vi "NMRvmefull7.vi"() -> ()   [LabVIEW 2013]
uses:
  <vilib>/Utility/file.llb/Read From Spreadsheet File (DBL).vi
  <vilib>/Analysis/NI_AALBase.lvlib
panel:
  out "Telnet error out":errorcluster
  in  "Real/quad Q curve":bool=TRUE
  out "Temperature (C)":dbl(graph)=23.38
  out "+3V supply":dbl=0.005 format="%_4g"
  out "Temp (C)":dbl=23.38 format="%_4g"
  in  "RemovePed":bool=TRUE
  in  "IF / LOG Det":bool
  in  "Q curve file":string="realback213.txt"
  out "File name 2":string="C:\\users\\plm\\Desktop\\rssmt\\realback213.txt"
  in  "AutoBaseline":bool=TRUE
  out "RF OK":bool=TRUE
  out "Peak area (V-MHz)":sgl=0.042041864 format="%.5f"
  in  "Gauss Fit":bool=TRUE
  out "NMR Graph + Fit":cluster{cluster{dbl, "Numeric":dbl}[]}[](graph)=[{[{212.6, "Numeric"=-0.015064761904761914}, {212.60999999999999, "Numeric"=0.0068132738095046524}, {212.62, "Numeric"=-0.005688690476169475}, {212.63, "Numeric"=0.007429345238097601}, {212.64, "Numeric"=0.00206738095236568}, {212.65, "Numeric"=0.0025254166666881794}, {212.66, "Numeric"=0.006503452380956669}, {212.67, "Numeric"=0.004701488095226254}, {212.68, "Numeric"=0.009119523809545282}, {212.69, "Numeric"=-0.0037424404761845914}, {212.7, "Numeric"=0.008815595238086477}, {212.71, "Numeric"=0.0006936309524021023}, {212.72, "Numeric"=0.006691666666673632}, {212.73, "Numeric"=0.008509702380946275}, {212.74, "Numeric"=0.0017477380952147722}, {212.75, "Numeric"=0.0074057738095315365}, {212.76, "Numeric"=-0.0027161904761943204}, {212.77, "Numeric"=0.007581845238075695}, {212.78, "Numeric"=-0.004200119047610973}, {212.79, "Numeric"=0.005137916666664702}, {212.8, "Numeric"=-0.011404047619063787}, {212.81, "Numeric"=-0.01402601190475386}, {212.82, "Numeric"=-0.012227976190476678}, {212.82999999999998, "Numeric"=0.005190059523801537}, {212.84, "Numeric"=-0.00597190476189715}, {212.85, "Numeric"=-0.015713869047618456}, {212.85999999999999, "Numeric"=-0.00983583333333872}, {212.87, "Numeric"=-0.00833779761904085}, {212.88, "Numeric"=-0.005119761904760638}, {212.89, "Numeric"=0.006818273809520627}, {212.9, "Numeric"=-0.004623690476184925}, {212.91, "Numeric"=-0.0011456547619032031}, {212.92, "Numeric"=0.0019523809523795694}, {212.93, "Numeric"=0.021770416666670588}, {212.94, "Numeric"=0.021808452380953823}, {212.95, "Numeric"=0.05906648809523813}, {212.96, "Numeric"=0.11614452380952572}, {212.97, "Numeric"=0.2472425595238105}, {212.98, "Numeric"=0.4608605952380963}, {212.99, "Numeric"=0.47679863095237796}, {213.0, "Numeric"=0.3593566666666667}, {213.01, "Numeric"=0.31613470238095404}, {213.02, "Numeric"=0.30183273809523725}, {213.03, "Numeric"=0.22655077380952257}, {213.04, "Numeric"=0.2235888095238114}, {213.05, "Numeric"=0.23714684523809612}, {213.06, "Numeric"=0.208224880952378}, {213.07, "Numeric"=0.24872291666666835}, {213.08, "Numeric"=0.2025409523809546}, {213.09, "Numeric"=0.13657898809523306}, {213.1, "Numeric"=0.07963702380952496}, {213.11, "Numeric"=0.06781505952381271}, {213.12, "Numeric"=0.04841309523808776}, {213.13, "Numeric"=0.03103113095238112}, {213.14000000000001, "Numeric"=0.0213691666666704}, {213.15, "Numeric"=0.0067272023809420226}, {213.16, "Numeric"=0.004605238095236934}, {213.17000000000002, "Numeric"=0.03380327380952772}, {213.18, "Numeric"=0.04402130952379589}, {213.19, "Numeric"=0.014959345238092323}, {213.2, "Numeric"=0.012717380952389792}, {213.21, "Numeric"=0.00889541666664935}, {213.22, "Numeric"=-0.0021065476190526844}, {213.23, "Numeric"=-0.008588511904753703}, {213.24, "Numeric"=-0.02205047619045882}, {213.25, "Numeric"=-0.010992440476198108}, {213.26, "Numeric"=-0.030914404761897572}, {213.27, "Numeric"=-0.016216369047601147}, {213.28, "Numeric"=-0.028298333333343903}, {213.29, "Numeric"=-0.021760297619041885}, {213.3, "Numeric"=-0.015602261904743953}, {213.31, "Numeric"=-0.0199242261904901}, {213.32, "Numeric"=-0.00022619047618652188}, {213.33, "Numeric"=-0.005708154761887109}, {213.34, "Numeric"=0.0072298809523633}, {213.35, "Numeric"=-0.009612083333331578}, {213.36, "Numeric"=-0.0036340476190306475}, {213.37, "Numeric"=0.004763988095216332}, {213.38, "Numeric"=0.009782023809522991}, {213.39000000000001, "Numeric"=0.021320059523825388}, {213.4, "Numeric"=0.016278095238068974}]}, {[{212.6, "Numeric"=5.584531821965065e-19}, {212.60999999999999, "Numeric"=3.978014328960224e-18}, {212.62, "Numeric"=2.700482036449847e-17}, {212.63, "Numeric"=1.7470752797417705e-16}, {212.64, "Numeric"=1.077152815916244e-15}, {212.65, "Numeric"=6.329048153969349e-15}, {212.66, "Numeric"=3.5440093194235226e-14}, {212.67, "Numeric"=1.8912401840252364e-13}, {212.68, "Numeric"=9.618202027801922e-13}, {212.69, "Numeric"=4.6616158273777845e-12}, {212.7, "Numeric"=2.1531507656689395e-11}, {212.71, "Numeric"=9.47780519405207e-11}, {212.72, "Numeric"=3.975909513227806e-10}, {212.73, "Numeric"=1.589500182399966e-09}, {212.74, "Numeric"=6.055918875558694e-09}, {212.75, "Numeric"=2.1988463950004145e-08}, {212.76, "Numeric"=7.608606280246018e-08}, {212.77, "Numeric"=2.5090580385633865e-07}, {212.78, "Numeric"=7.88518123558403e-07}, {212.79, "Numeric"=2.3616091812368746e-06}, {212.8, "Numeric"=6.740618590002307e-06}, {212.81, "Numeric"=1.8335250824726833e-05}, {212.82, "Numeric"=4.753016626889281e-05}, {212.82999999999998, "Numeric"=0.00011742138213886348}, {212.84, "Numeric"=0.00027645243462944805}, {212.85, "Numeric"=0.0006202817826469859}, {212.85999999999999, "Numeric"=0.0013263343280559513}, {212.87, "Numeric"=0.0027027904165697262}, {212.88, "Numeric"=0.005248885595362881}, {212.89, "Numeric"=0.009714427693085783}, {212.9, "Numeric"=0.017134155719277566}, {212.91, "Numeric"=0.02880073528497979}, {212.92, "Numeric"=0.046135987189811954}, {212.93, "Numeric"=0.0704322295945597}, {212.94, "Numeric"=0.10247040006473142}, {212.95, "Numeric"=0.1420760267927174}, {212.96, "Numeric"=0.18773210570032461}, {212.97, "Numeric"=0.2364022882231464}, {212.98, "Numeric"=0.28370054939484945}, {212.99, "Numeric"=0.3244621593392298}, {213.0, "Numeric"=0.3536415683173779}, {213.01, "Numeric"=0.3673313019215627}, {213.02, "Numeric"=0.3636201525459477}, {213.03, "Numeric"=0.3430309670843958}, {213.04, "Numeric"=0.30839979958758623}, {213.05, "Numeric"=0.26423492712989627}, {213.06, "Numeric"=0.21575543037604758}, {213.07, "Numeric"=0.1678914670658022}, {213.08, "Numeric"=0.12450617443201661}, {213.09, "Numeric"=0.08799308229736456}, {213.1, "Numeric"=0.059265444880766016}, {213.11, "Numeric"=0.038040826422342765}, {213.12, "Numeric"=0.02326985698277657}, {213.13, "Numeric"=0.013565408032532578}, {213.14000000000001, "Numeric"=0.007536459768259726}, {213.15, "Numeric"=0.0039902240808005794}, {213.16, "Numeric"=0.002013365218657428}, {213.17000000000002, "Numeric"=0.0009681512595222955}, {213.18, "Numeric"=0.0004436691628551842}, {213.19, "Numeric"=0.00019376291080760256}, {213.2, "Numeric"=8.064499741229013e-05}, {213.21, "Numeric"=3.1987447860996285e-05}, {213.22, "Numeric"=1.2091414969278342e-05}, {213.23, "Numeric"=4.355821133391314e-06}, {213.24, "Numeric"=1.4954032687879686e-06}, {213.25, "Numeric"=4.892625674974261e-07}, {213.26, "Numeric"=1.5255309774177953e-07}, {213.27, "Numeric"=4.5331015490803665e-08}, {213.28, "Numeric"=1.2837050265778443e-08}, {213.29, "Numeric"=3.4644190009270176e-09}, {213.3, "Numeric"=8.910271930804879e-10}, {213.31, "Numeric"=2.1839710707625631e-10}, {213.32, "Numeric"=5.1015034032640396e-11}, {213.33, "Numeric"=1.1356509185476955e-11}, {213.34, "Numeric"=2.4092779655767407e-12}, {213.35, "Numeric"=4.871069626718068e-13}, {213.36, "Numeric"=9.385494131204198e-14}, {213.37, "Numeric"=1.7233969657075795e-14}, {213.38, "Numeric"=3.0158440610570367e-15}, {213.39000000000001, "Numeric"=5.029534786345766e-16}, {213.4, "Numeric"=7.993594748403543e-17}]}]
  in  "Amp of Q curve":dbl=2.9 min=0.0 max=7.0 step=0.01 format="%_3f"
  in  "Subtract Q curve":bool=TRUE
  in  "Adjust Tune":bool
  out "Pedestal Offset":dbl(graph)=0.03187083333333342
  out "Pedestal Difference":dbl(graph)=0.10203000000000387
  out "# Good Spectra":i32=996
  in  "Quality cuts":bool=TRUE
  out "Pedestal OK":bool=TRUE
  out "Sweep #":i32=936
  out "1st Sweep":bool
  out "ADC volts OK":bool=TRUE
  out "Peak Height Distribution":cluster{"Y":dbl[], "Y":dbl[]}[](graph)=[{"Y"=[0.3583456394333454, 0.3587091757975026, 0.3590727121616598, 0.359436248525817, 0.35979978488997416, 0.36016332125413136, 0.36052685761828857, 0.36089039398244577, 0.36125393034660297, 0.36161746671076017, 0.3619810030749174, 0.3623445394390746, 0.3627080758032317, 0.3630716121673889, 0.3634351485315461, 0.36379868489570333, 0.36416222125986053, 0.36452575762401773, 0.36488929398817493, 0.3652528303523321, 0.3656163667164893, 0.3659799030806465, 0.3663434394448037, 0.3667069758089609, 0.3670705121731181, 0.3674340485372753, 0.3677975849014325, 0.36816112126558964, 0.36852465762974684, 0.36888819399390405, 0.36925173035806125, 0.36961526672221845, 0.36997880308637565, 0.37034233945053285, 0.37070587581469006, 0.3710694121788472, 0.3714329485430044, 0.3717964849071616, 0.3721600212713188, 0.372523557635476, 0.3728870939996332, 0.3732506303637904, 0.37361416672794756, 0.37397770309210476, 0.37434123945626196, 0.37470477582041917, 0.37506831218457637, 0.37543184854873357, 0.3757953849128908, 0.376158921277048, 0.3765224576412051, 0.3768859940053623, 0.3772495303695195, 0.3776130667336767, 0.37797660309783393, 0.37834013946199113, 0.37870367582614833, 0.37906721219030554, 0.3794307485544627, 0.3797942849186199, 0.3801578212827771, 0.3805213576469343, 0.3808848940110915, 0.3812484303752487, 0.3816119667394059, 0.38197550310356304, 0.38233903946772024, 0.38270257583187745, 0.38306611219603465, 0.38342964856019185, 0.38379318492434905, 0.38415672128850625, 0.38452025765266346, 0.3848837940168206, 0.3852473303809778, 0.385610866745135, 0.3859744031092922, 0.3863379394734494, 0.3867014758376066, 0.3870650122017638, 0.387428548565921, 0.38779208493007816, 0.38815562129423536, 0.38851915765839257, 0.38888269402254977, 0.38924623038670697, 0.3896097667508642, 0.3899733031150214, 0.3903368394791786, 0.3907003758433357, 0.3910639122074929, 0.3914274485716501, 0.39179098493580733, 0.39215452129996453, 0.39251805766412173, 0.39288159402827894, 0.3932451303924361, 0.3936086667565933, 0.3939722031207505, 0.3943357394849077], "Y"=[1.0, 0.0, 0.0, 0.0, 0.0, 1.0, 1.0, 2.0, 5.0, 1.0, 2.0, 1.0, 1.0, 4.0, 4.0, 4.0, 3.0, 3.0, 5.0, 4.0, 4.0, 5.0, 6.0, 8.0, 6.0, 8.0, 5.0, 10.0, 9.0, 12.0, 17.0, 21.0, 14.0, 12.0, 14.0, 26.0, 16.0, 20.0, 24.0, 27.0, 24.0, 22.0, 20.0, 27.0, 17.0, 30.0, 32.0, 22.0, 21.0, 25.0, 26.0, 20.0, 14.0, 20.0, 16.0, 16.0, 18.0, 18.0, 22.0, 23.0, 13.0, 15.0, 15.0, 11.0, 13.0, 14.0, 15.0, 11.0, 9.0, 9.0, 13.0, 12.0, 7.0, 10.0, 14.0, 8.0, 5.0, 4.0, 4.0, 5.0, 3.0, 6.0, 4.0, 1.0, 2.0, 4.0, 2.0, 2.0, 5.0, 3.0, 0.0, 3.0, 3.0, 3.0, 2.0, 1.0, 3.0, 1.0, 0.0, 2.0]}]
  in  "# of Sweeps":i32=1000
  out "Std Dev (V)":dbl=0.006381391256445841 format="%_2g"
  out "Peak mean (V)":dbl=0.3761242600279397 format="%_4g"
  out "Peak Height":dbl(graph)=0.3680706435940542
  in  "Raw Data":bool=TRUE
  in  "Tank RF":bool=TRUE
  in  "IF Atten (dB)":i8 min=0 max=31 step=1
  in  "IFoffset (V)":dbl=-2.0946619999999916 min=-4.0 max=4.0 step=0.001 format="%.4f"
  in  "Tune  (V)":dbl=0.6173 min=0.0 max=5.0 step=0.001 format="%.4f"
  in  "Hi / Lo IF Gain":bool
  out "Voltage Array":sgl[](array[numeric])=[0.4196, 0.4201, 0.3868, 0.3797, 0.3547, 0.3361, 0.3216, 0.3019, 0.289, 0.2594, 0.2558, 0.2321, 0.2231, 0.2105, 0.1899, 0.1823, 0.1595, 0.1577, 0.1344, 0.1328, 0.1059, 0.0935, 0.0861, 0.0949, 0.0757, 0.0585, 0.0575, 0.0527, 0.0502, 0.057, 0.041, 0.0405, 0.0402, 0.0572, 0.055, 0.0906, 0.1466, 0.2772, 0.4909, 0.5075, 0.3913, 0.3499, 0.338, 0.2657, 0.2663, 0.284, 0.2598, 0.3056, 0.2653, 0.2058, 0.1559, 0.1517, 0.1405, 0.1319, 0.1316, 0.1269, 0.1353, 0.1756, 0.1975, 0.1807, 0.1913, 0.2009, 0.2039, 0.212, 0.2137, 0.2405, 0.2369, 0.2685, 0.2739, 0.2985, 0.3233, 0.3382, 0.3777, 0.3926, 0.4265, 0.4312, 0.4593, 0.4904, 0.5187, 0.5541, 0.5735] format="%.4f"
  in  "Invert Polarity":bool
  out "Pedestal Diff (V)":sgl=0.10203 format="%.3f"
  out "Peak amp (V)":sgl=0.36807063 format="%.3f"
  in  "Save Data to File":bool
  in  "RF Level (dBm)":dbl=-1.0 min=-10.0 max=10.0 step=0.1 format="%.2f"
  out "SMT error out":errorcluster
  out "Sample RMS (V)":dbl=0.01354814814814815 format="%.4f"
  in  "# Sample/step":i32=80 min=1 max=1000 step=100
  in  "Step Width (MHz)":dbl=0.01 min=0.0 max=1000.0 step=0.0005 format="%.4f"
  in  "Freq Span (MHz)":dbl=0.8 min=0.0 max=3000.0 step=0.1 format="%.3f"
  in  "Center Freq (MHz)":dbl=213.0 min=0.005 max=6000.0 step=0.1 format="%.3f"
  in  "Sweep Mode":u16(ring)=3 items=["Off", "Single", "Auto", "Step"]
  in  "GPIB Addr (28)":refnum<visa-resource-name>="GPIB0::28::INSTR"
  # "E1039 Prototype NMR Control Panel"
  # "Settings"
  # "D\nA\nC"
  # "R\nF\n\nG\nE\nN \n\n+\n\nI\nF"
  # "A\nD\nC"
  # "D\nA\nT\nA\n\n+\n\nA \nN\nA\nL\nY\nS\nI\nS"
  # "I\n/\nO"
  # "Results"
  # "A\nv\ne\nr\na\ng\ne"
  # "S\nw\ne\ne\np"
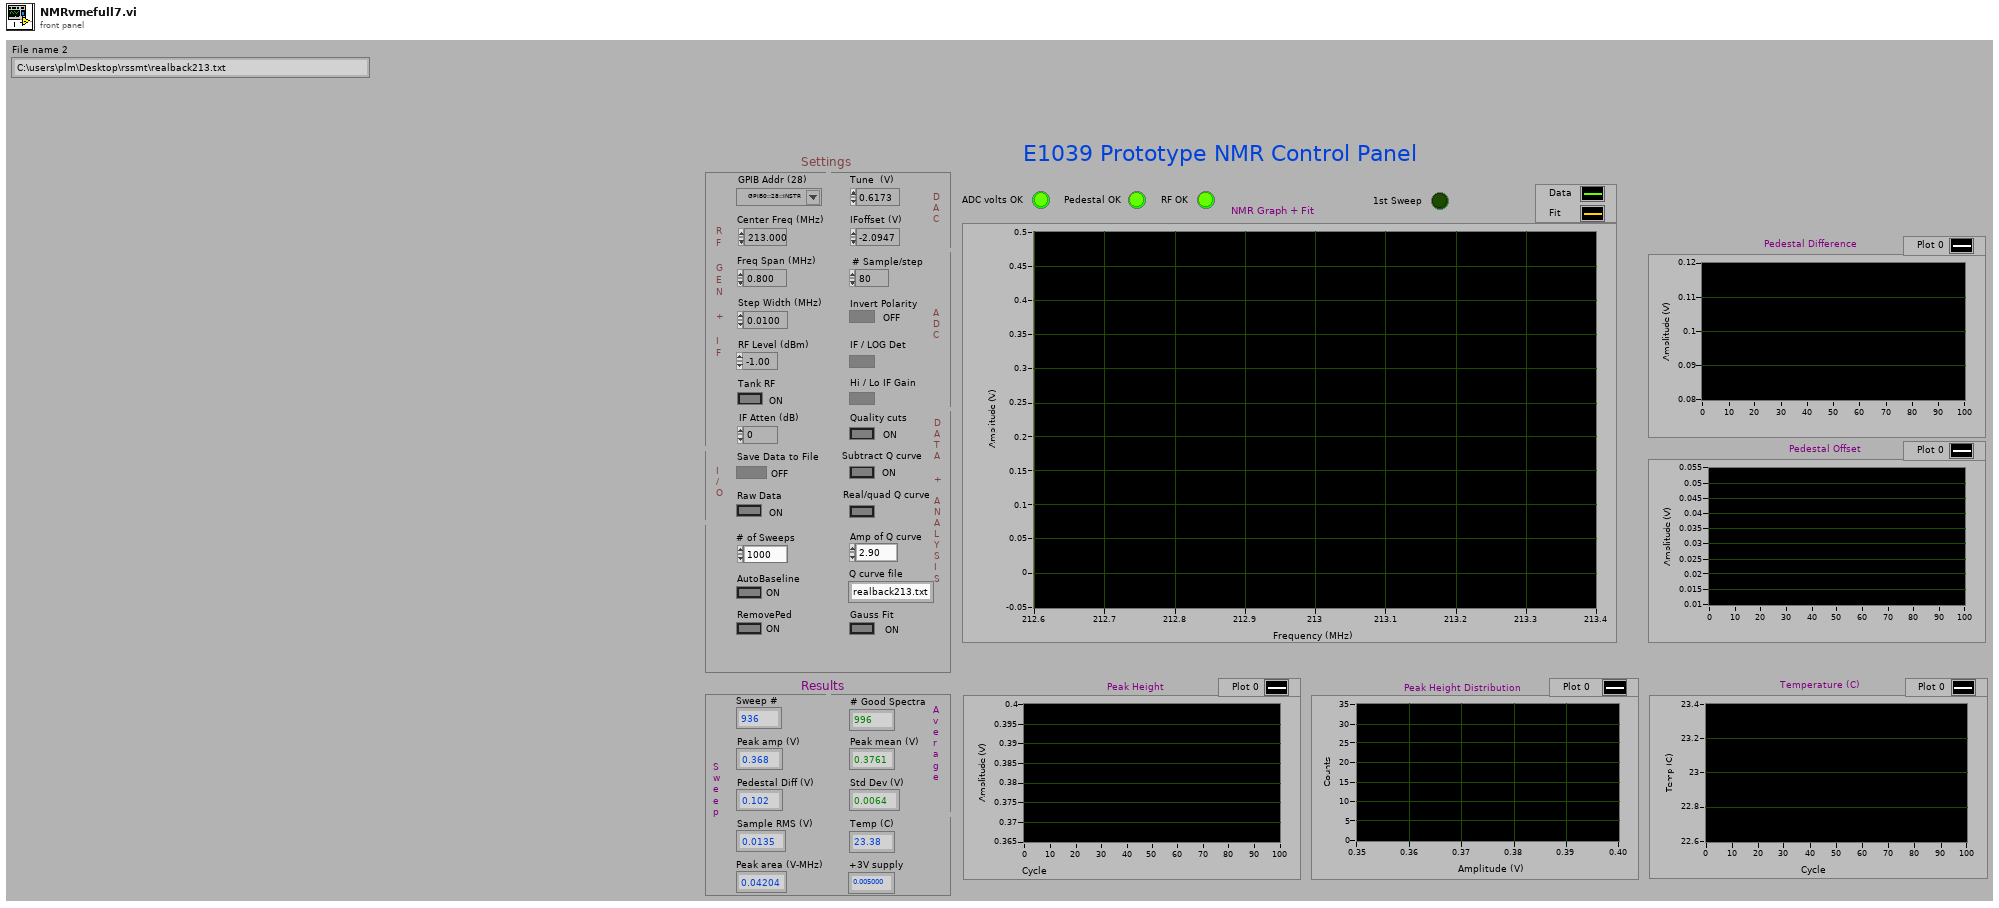
[diagram p1: front panel]
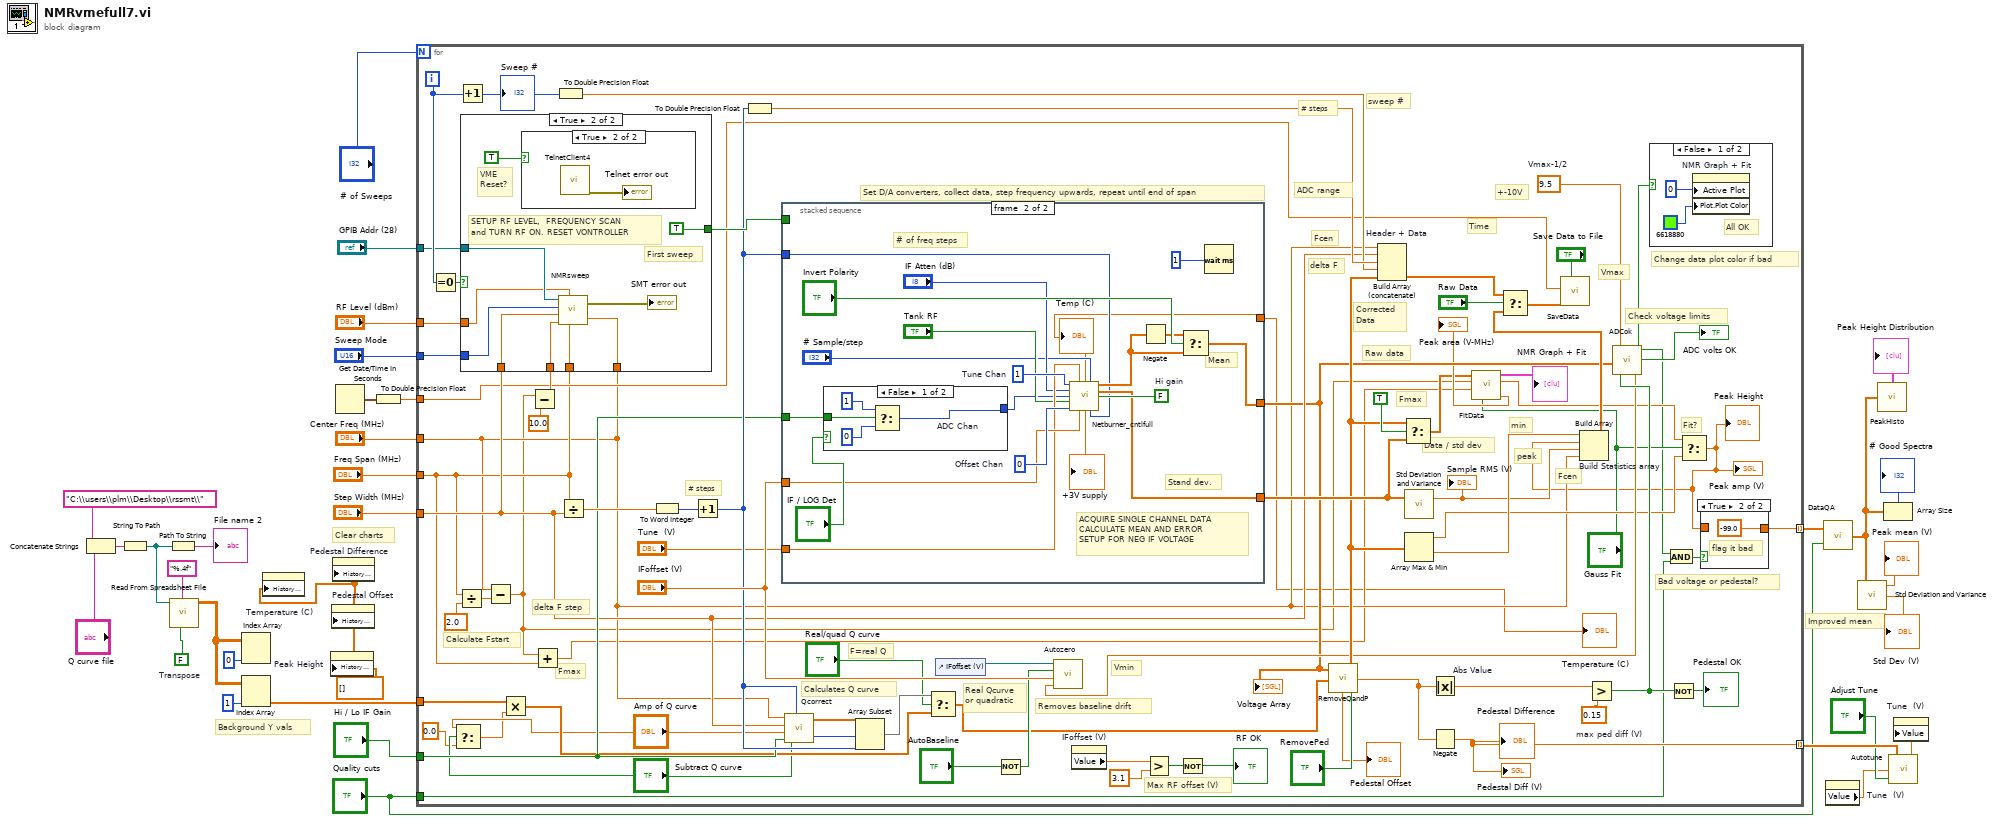
[diagram p0: block diagram]
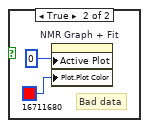
[diagram p2: hidden frame]
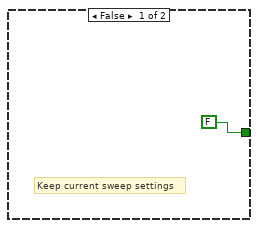
[diagram p4: hidden frame]
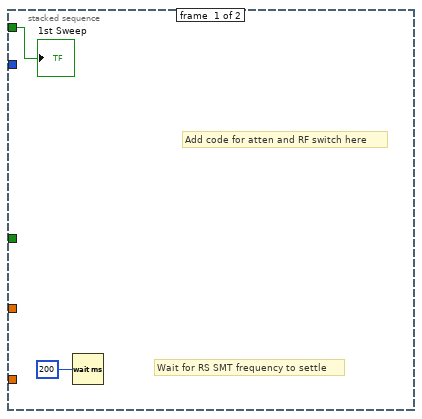
[diagram p6: hidden frame]
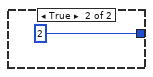
[diagram p7: hidden frame]
diagram:
  w9 = FALSE  # Transpose
  w1 = dbl[] []
  # "Background Y vals"
  # "Clear charts"
  # "Improved mean"
  n1 = Concatenate Strings "Concatenate Strings"("C:\\users\\plm\\Desktop\\rssmt\\", "Q curve file") -> (w12:string)
  n2 = String To Path(string=w12) -> (path=w8:path)
  n3 = Path To String(path=w8) -> (string=→"File name 2":string)
  n4 = call-poly <vilib>:"Read From Spreadsheet File.vi"("transpose (no:F)"=w9, "format (%.3f)"="%.4f", "file path (dialog if empty)"=w8) -> ("all rows"=w7:dbl[][])  [unwired: 4 in, 4 out]
  n5 = Index Array "Index Array"(array=w7, index (col)=0) -> ()  [unwired: 1 in, 1 out]
  n6 = Index Array(array=w7, index (col)=1) -> (element=w2:dbl[])  [unwired: 1 in]
  n7 = property on="Temperature (C)" class="WFChart (strict)"("History Data"=w1) -> ()  [unwired: 2 in, 2 out]
  n8 = property on="Peak Height" class="WFChart (strict)"("History Data"=w1) -> ()  [unwired: 2 in, 2 out]
  n9 = property on="Pedestal Offset" class="WFChart (strict)"("History Data"=w1) -> ()  [unwired: 2 in, 2 out]
  n10 = property on="Pedestal Difference" class="WFChart (strict)"("History Data"=w1) -> ()  [unwired: 2 in, 2 out]
  n11 = Get Date/Time In Seconds() -> (seconds since 1Jan1904=w14:timestamp)
  n12 = To Double Precision Float(number=w14) -> (double precision float=w13:dbl)
  n13 = for {
    N: "# of Sweeps" -> [_]
    tunnel: [w94] -> w29 mode=indexing
    tunnel: "Quality cuts" -> [w71]
    tunnel: [w77] -> w26 mode=indexing
    tunnel: "Center Freq (MHz)" -> [w58]
    tunnel: "Freq Span (MHz)" -> [w64]
    tunnel: "Step Width (MHz)" -> [w70]
    tunnel: "Sweep Mode" -> [w81]
    tunnel: "Hi / Lo IF Gain" -> [w80]
    tunnel: "GPIB Addr (28)" -> [w79]
    tunnel: "RF Level (dBm)" -> [w78]
    tunnel: w13 -> [w65]
    tunnel: w2 -> [w43]
    i -> [w92]
    w75 = 9.5  # Vmax-1/2
    w95 = 0.15  # max ped diff (V)
    # "F=real Q"
    # "Real Qcurve\nor quadratic"
    # "+-10V"
    # "Vmax"
    # "Change data plot color if bad"
    # "Max RF offset (V)"
    # "Fmax"
    # "Fit?"
    # "Fmax"
    # "Time"
    # "Vmin"
    # "min"
    # "peak"
    # "Raw data"
    # "Corrected\nData"
    # "Fcen"
    # "delta F"
    # "# steps"
    # "ADC range"
    # "sweep #"
    # "Fcen"
    # "Set D/A converters, collect data, step frequency upwards, repeat until end of span"
    # "Calculates Q curve"
    # "Removes baseline drift"
    # "Bad voltage or pedestal?"
    # "Check voltage limits"
    # "Data / std dev"
    # "# steps"
    # "Calculate Fstart"
    # "delta F step"
    n14 = Equal To 0?(x=w92) -> (x = 0?=w97:bool)
    n15 = Select(t="Amp of Q curve", s="Subtract Q curve", f=0.0) -> (s? t:f=w38:dbl)
    n16 = Divide(x=w64, y=sgl 2.0) -> (x/y=w108:dbl)
    n17 = Increment(x=w92) -> (x+1=w82:i32)
    "Sweep #" <- w82
    n18 = Subtract(x=w58, y=w108) -> (x-y=w53:dbl)
    n19 = Multiply(x=w43, y=w38) -> (x*y=w42:dbl[])
    n20 = Subtract(x=w53, y=10.0) -> (x-y=w106:dbl)
    n21 = case shown="True" w97 {
      tunnel: w106 -> [_ w127]
      tunnel: w70 -> [_ w125]
      tunnel: w58 -> [_ w124]
      tunnel: w64 -> [_ w126]
      tunnel: [FALSE TRUE] -> w96
      tunnel: w81 -> [_ w121]
      tunnel: w79 -> [_ w120]
      tunnel: w78 -> [_ w119]
      frame False {
        # "Keep current sweep settings"
      }
      frame True {
        # "VME\nReset?"
        # "First sweep"
        # "SETUP RF LEVEL,  FREQUENCY SCAN\nand TURN RF ON. RESET VONTROLLER"
        n22 = case shown="True" TRUE {
          frame False {
          }
          frame True {
            n23 = call "TelnetClient4.vi"() -> ("Telnet error"=→"Telnet error out":errorcluster)  [unwired: 4 in, 3 out]
          }
        }
        n24 = call "NMRsweep.vi"("Center Freq (MHz)"=w124, "Freq Span (MHz)"=w126, "RF Level (dBm)"=w119, "Foffset (MHz)"=w127, "Step Width (MHz)"=w125, "Sweep Mode"=w121, "GPIB Addr (28)"=w120) -> ("error out"=→"SMT error out":errorcluster)
      }
    }
    n25 = Add(x=w53, y=w64) -> (x+y=w52:dbl)
    n26 = To Double Precision Float(number=w82) -> (double precision float=w83:dbl)
    n27 = Divide(x=w64, y=w70) -> (x/y=w110:dbl)
    n28 = To Word Integer(number=w110) -> (16bit integer=w107:i16)
    n29 = Increment(x=w107) -> (x+1=w86:i16)
    n30 = To Double Precision Float(number=w86) -> (double precision float=w85:dbl)
    n31 = stacked-sequence {
      tunnel: [_ w136] -> w100
      tunnel: [_ w148] -> w68
      tunnel: w86 -> [_ w133]
      tunnel: "IFoffset (V)" -> [_ w143]
      tunnel: w80 -> [_ w146]
      tunnel: w96 -> [w129 _]
      tunnel: "Tune  (V)" -> [_ w141]
      tunnel: [_ w131] -> w34
      frame #0 {
        # "Add code for atten and RF switch here"
        # "Wait for RS SMT frequency to settle"
        n32 = Wait (ms)(milliseconds to wait=200) -> ()  [unwired: 1 out]
        "1st Sweep" <- w129
      }
      frame #1 {
        w138 = FALSE  # Hi gain
        w144 = 0  # Offset Chan
        w142 = 1  # Tune Chan
        # "Stand dev."
        # "Mean"
        # "ACQUIRE SINGLE CHANNEL DATA\nCALCULATE MEAN AND ERROR\nSETUP FOR NEG IF VOLTAGE"
        # "# of freq steps"
        n33 = case shown="False" "IF / LOG Det" {
          tunnel: w146 -> [w154 _]
          tunnel: [w151 2] -> w135
          frame False {
            n34 = Select "ADC Chan"(t=1, s=w154, f=0) -> (s? t:f=w151:i32)
          }
          frame True {
          }
        }
        n35 = call "Netburner_cntlfull.vi"("Tune DAC"=w142, "Tune Volt"=w141, "# Data"="# Sample/step", "IF Atten (dB)"="IF Atten (dB)", "NMR ADC"=w135, "Hi Gain"=w138, "Tank RF"="Tank RF", "Offset DAC"=w144, "Offset Volt"=w143, "# f steps"=w133) -> ("Temp (C)"=w131:dbl, "ADC value"=w137:dbl[], "ADC error"=w136:dbl[], "Volts"=→"+3V supply":dbl)  [unwired: 2 out]
        "Temp (C)" <- w131
        n36 = Negate(x=w137) -> (-x=w147:dbl[])
        n37 = Select(t=w147, s="Invert Polarity", f=w137) -> (s? t:f=w148:dbl[])
        n38 = Wait (ms)(milliseconds to wait=1) -> ()  [unwired: 1 out]
      }
    }
    "Voltage Array" <- w68
    "Temperature (C)" <- w34
    n39 = call "Qcorrect.vi"("Subtract Q curve"="Subtract Q curve", "Nstep"=w86, "IF or Log"=w80, "Amp of Q curve"="Amp of Q curve", "Step Width (MHz)"=w70, "Center Freq (MHz)"=w58) -> ("Start"=w101:i32, "Array"=w102:dbl[])
    n40 = Array Subset "Array Subset"(array=w102, index=w101, length=w86) -> (w46:dbl[])
    n41 = Select(t=w46, s="Real/quad Q curve", f=w42) -> (s? t:f=w45:dbl[])
    n42 = control-ref of="IFoffset (V)"() -> (w74:refnum<vi>)
    n43 = Not(x="AutoBaseline") -> (.not. x?=w47:bool)
    n44 = property on="IFoffset (V)" class="DigNum (strict)"() -> ("Value"=w62:dbl)  [unwired: 2 in, 2 out]
    n45 = Greater?(x=w62, y=3.1) -> (0:w60:bool)
    n46 = Not(x=w60) -> (.not. x?=→"RF OK":bool)
    n47 = call "RemoveQandP.vi"("Subtract Ped?"="RemovePed", "Qcurve"=w45, "Raw data"=w68) -> ("Ped L-R"=w88:dbl, "Corrected data"=w84:dbl[], "Ped Offfset"=→"Pedestal Offset":dbl)
    n48 = Build Array (concatenate) "Header + Data"(w58, w70, w85, w83, w84) -> (w87:dbl[])
    n49 = Select(t=w84, s=TRUE, f=w100) -> (s? t:f=w54:dbl[])
    n50 = call <vilib>:"Std Deviation and Variance.vi"("X"=w100) -> ("mean"=w69:dbl)  [unwired: 1 in, 2 out]
    "Sample RMS (V)" <- w69
    n51 = Array Max & Min(array=w84) -> (max value=w63:dbl, min value=w99:dbl)  [unwired: 2 out]
    n52 = Absolute Value "Abs Value"(x=w88) -> (abs(x)=w90:dbl)
    n53 = Negate(x=w88) -> (-x=w77:dbl)
    "Pedestal Diff (V)" <- w77
    "Pedestal Difference" <- w77
    n54 = call "FitData.vi"("Fit?"="Gauss Fit", "Fmax"=w52, "Fmin"=w53, "Yarray"=w54) -> ("Peak Area (V-MHz)"=→"Peak area (V-MHz)":dbl, "Amplitude (V)"=w56:dbl, "NMR Graph + Fit"=→"NMR Graph + Fit":cluster{cluster{dbl, "Numeric":dbl}[]}[])  [unwired: 2 out]
    n55 = Greater?(x=w90, y=w95) -> (0:w76:bool)
    n56 = call "ADCok.vi"("PedOK"=w76, "Array"=w68, "Vmax-1/2"=w75) -> ("Vmin"=w73:dbl, "ADC voltages OK"=→"ADC volts OK":bool, "Allok"=w50:bool)
    n57 = call "Autozero.vi"("Vmin (V)"=w73, "IFoffset (V)"="IFoffset (V)", "IF or Log"=w47, "reference"=w74) -> ()
    n58 = case shown="False" w50 {
      frame False {
        # "All OK"
        n59 = property on="NMR Graph + Fit" class="XYGraph (strict)"("Active Plot"=0, "Plot.Plot Color"=u32 6618880) -> ()  [unwired: 2 in, 2 out]
      }
      frame True {
        # "Bad data"
        n60 = property on="NMR Graph + Fit" class="XYGraph (strict)"("Active Plot"=0, "Plot.Plot Color"=u32 16711680) -> ()  [unwired: 2 in, 2 out]
      }
    }
    n61 = And(x=w50, y=w71) -> (x .and. y?=w91:bool)
    n62 = Not(x=w76) -> (.not. x?=→"Pedestal OK":bool)
    n63 = Select(t=w56, s="Gauss Fit", f=w63) -> (s? t:f=w49:dbl)
    "Peak amp (V)" <- w49
    "Peak Height" <- w49
    n64 = Build Array "Build Statistics array"(w99, w49, w69, w58) -> (w105:dbl[])
    n65 = Select(t=w87, s="Raw Data", f=w105) -> (s? t:f=w66:dbl[])
    n66 = call "SaveData.vi"("Array"=w66, "Save Data to File"="Save Data to File", "Ext time (sec)"=w65) -> ()  [unwired: 1 out]
    n67 = case shown="True" w91 {
      tunnel: [w115 -99.0] -> w94
      tunnel: w49 -> [w115 _]
      frame False {
        # "Data OK"
      }
      frame True {
        # "flag it bad"
      }
    }
  }
  n68 = call "DataQA.vi"("Quality cuts"="Quality cuts", "Data In"=w29) -> ("Data Out"=w28:dbl[])
  n69 = property on="Tune  (V)" class="DigNum (strict)"() -> ("Value"=w17:dbl)  [unwired: 2 in, 2 out]
  n70 = call <vilib>:"Std Deviation and Variance.vi"("X"=w28) -> ("mean"=→"Peak mean (V)":dbl, "standard deviation"=→"Std Dev (V)":dbl)  [unwired: 1 in, 1 out]
  n71 = call "PeakHisto.vi"("Data Out"=w28) -> ("XY Graph"=→"Peak Height Distribution":cluster{"Y":dbl[], "Y":dbl[]}[])
  n72 = Array Size(array=w28) -> (size(s)=→"# Good Spectra":i32)
  n73 = call "Autotune.vi"("Adjust Tune"="Adjust Tune", "Tune Vin"=w17, "Pedestal Diff"=w26) -> ("Tune Vout"=w16:dbl)
  n74 = property on="Tune  (V)" class="DigNum (strict)"("Value"=w16) -> ()  [unwired: 2 in, 2 out]
